vi "Get SMO Base Events.vi"(8 "error in (no error)":errorcluster, 11 "PublicEvents in":refnum<class "PublicEvents.lvclass">) -> (0 "error out":errorcluster, 2 "SMO Base Events":T1, 3 "PublicEvents out":refnum<class "PublicEvents.lvclass">)   [LabVIEW 2013, in "PublicEvents.lvclass"]
uses:
  PublicEvents.lvclass
  SMO/Typedefs/Public Events.ctl
  SMO/Typedefs/SMOState --Enum.ctl
  SMO/Typedefs/Reserve State--Enum.ctl
  PublicEvents.lvclass/PublicEvents.ctl
  SMO/SMO.lvclass
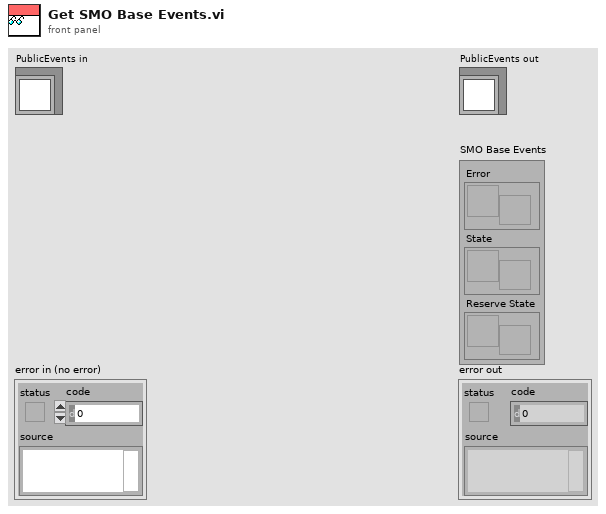
[diagram p1: front panel]
types:
  T1 = typedef "SMO.lvclass/Public Events.ctl" = cluster{"Error":refnum<user-event>, "State":refnum<user-event>, "Reserve State":refnum<user-event>}
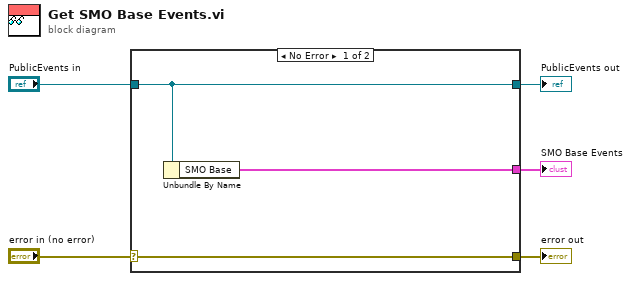
[diagram p0: block diagram]
diagram:
  n1 = case shown="No Error" "error in (no error)" {
    selector: "error in (no error)" -> [w8 w9]
    tunnel: [w8 w9] -> w4
    tunnel: [w7 w10] -> w2
    tunnel: "PublicEvents in" -> [w7 w10]
    tunnel: [w6 _] -> w1
    frame No Error {
      n2 = Unbundle By Name(w7) -> ("SMO Base"=w6:T1)
    }
    frame Error {
    }
  }
  "error out" <- w4
  "PublicEvents out" <- w2
  "SMO Base Events" <- w1
